vi "Build.vi"   [LabVIEW 2017, in "Scripts.lvlib"]
doc: "Builds all of the build specifications defined in this project."
uses:
  Scripts.lvlib
  <vilib>/AppBuilder/AB_API_Simple/Build (path).vi
  <vilib>/AppBuilder/AB_API_Simple/NI_App_Builder_API.lvlib
panel:
  # "Overview: Builds all Source Distribution specifications for this project\nRequirements: LabVIEW\nInstructions: Run this VI.\n\nThis VI builds all of the build specifications for this project. Any version of LabVIEW that supports projects and the Application Builder API can be used."
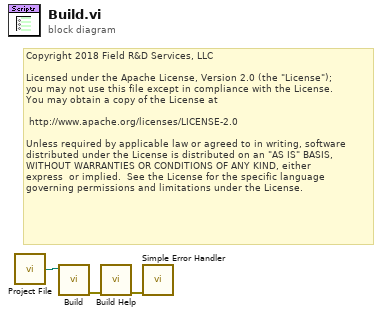
[diagram p0: block diagram]
diagram:
  # "Copyright 2018 Field R&D Services, LLC\n\nLicensed under the Apache License, Version 2.0 (the \"License\");\nyou may not use this file except in compliance with the License.\nYou may obtain a copy of the License at\n\n\thttp://www.apache.org/licenses/LICENSE-2.0\n\nUnless required by applicable law or agreed to in writing, software\ndistributed under the License is distributed on an \"AS IS\" BASIS,\nWITHOUT WARRANTIES OR CONDITIONS OF ANY KIND, either \nexpress  or implied.  See the License for the specific language \ngoverning permissions and limitations under the License."
  n1 = call "Project File.vi"() -> ("Project File"=w1:path)
  n2 = call-poly <vilib>:"Build.vi"("Path to project"=w1) -> ("error out"=w3:errorcluster)  [unwired: 9 in, 1 out]
  n3 = call "Build Help.vi"("Error In"=w3) -> ("Error Out"=w2:errorcluster)  [unwired: 9 in, 1 out]
  n4 = call <vilib>:"Simple Error Handler.vi"("error in (no error)"=w2) -> ()  [unwired: 4 in, 5 out]
